vi "CloseBaxterCamera.vi"(3 "error in":errorcluster, 4 "Camera":T1, 5 "node":string) -> (0 "error out":errorcluster, 1 "Error Code":i32, 2 "OK?":bool)   [LabVIEW 2012]
uses:
  <userlib>/ROSforLV/ROS/Code/SubVIs/BaxterCamera.ctl
  <userlib>/ROSforLV/ROS/Code/Console/Servers/ServerSubs/TopicDef.ctl
  <userlib>/ROSforLV/ROS/Code/SubVIs/_ROSDirection.ctl
  <userlib>/ROSforLV/ROS/MessageBuilding/std_msgs/subs/stringScalar.vi
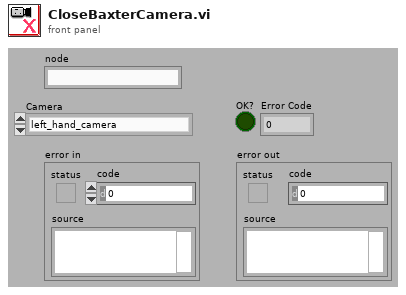
[diagram p1: front panel]
types:
  T1 = typedef "BaxterCamera.ctl" = enum16{"left_hand_camera", "right_hand_camera", "head_camera"}
  T2 = typedef "TopicDef.ctl" = cluster{"Topic":string, "Type":string, "Action":T3, "Update (ms)":u16, "write queue":u16}
  T3 = typedef "_ROSDirection.ctl" = enum16{"Node", "Publisher", "Subscriber", "Service Client"}
  T4 = typedef "_ROSControl.ctl" = cluster{"topic port":u16, "Node":string, "topic":string, "type":string, "node port":u16, "error ":errorcluster, "Direction":T3, "APIs":string[], "Update (ms)":u16, "write queue":u16}
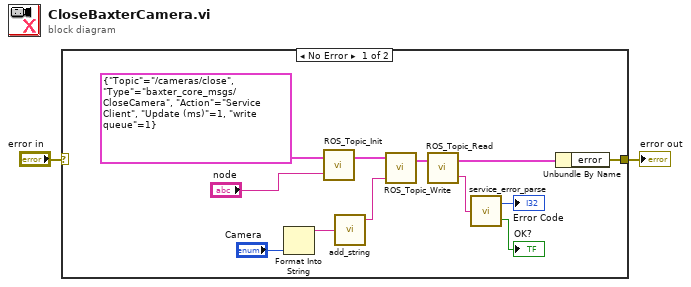
[diagram p0: block diagram]
diagram:
  n1 = case shown="No Error" "error in" {
    selector: "error in" -> [_ w15]
    tunnel: [w14 w15] -> w2
    frame No Error {
      n2 = Format Into String("Camera") -> (resulting string=w4:string)  [unwired: 3 in, 1 out]
      n3 = call <userlib>:"ROS_Topic_Init.vi"("node"="node", "Definitions"=T2 {"Topic"="/cameras/close", "Type"="baxter_core_msgs/CloseCamera", "Action"=enum."Service Client", "Update (ms)"=1, "write queue"=1}) -> ("ROS out"=w12:T4)  [unwired: 1 in]
      n4 = call-poly <userlib>:"add_string.vi"("String"=w4) -> ("msg out"=w6:string)  [unwired: 4 in]
      n5 = call <userlib>:"ROS_Topic_Write.vi"("Msg in"=w6, "ROS in"=w12) -> ("ROS out"=w11:T4)  [unwired: 2 in]
      n6 = call <userlib>:"ROS_Topic_Read.vi"("ROS in"=w11) -> ("Reply"=w9:string, "ROS out"=w10:T4)  [unwired: 1 in]
      n7 = call <userlib>:"service_error_parse.vi"("Reply"=w9) -> ("OK?"=→"OK?":bool, "Error Code"=→"Error Code":i32)
      n8 = Unbundle By Name(w10) -> ("error"=w14:errorcluster)
    }
    frame Error {
    }
  }
  "error out" <- w2
